vi "ChangePanel.vi"(8 "error in (no error)":errorcluster, 11 "Maui 2.0 in":refnum<class "Maui 2.0.lvclass">) -> (0 "error out":errorcluster, 3 "Maui 2.0 out":refnum<class "Maui 2.0.lvclass">)   [LabVIEW 2020, in "Maui 2.0.lvclass"]
uses:
  Maui 2.0.lvclass
panel:
  in  "Value":i32
  in  "Panel":i32
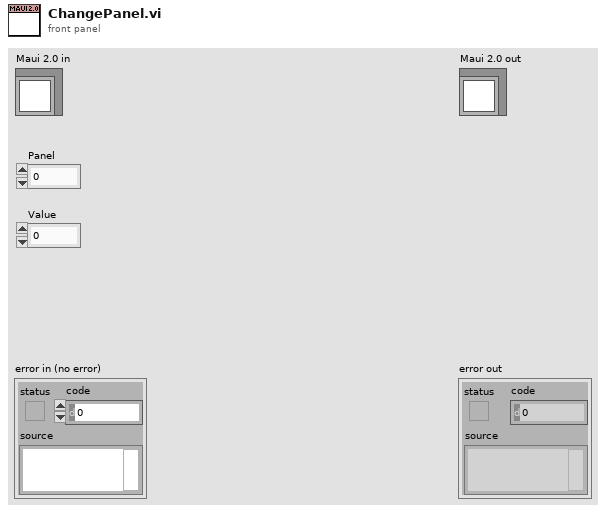
[diagram p1: front panel]
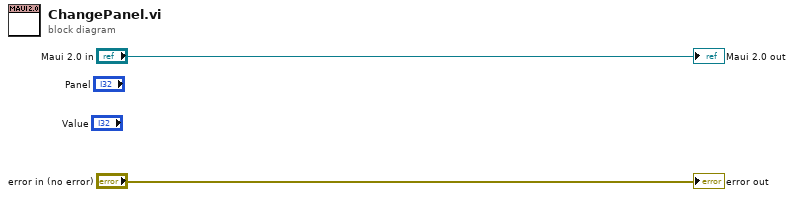
[diagram p0: block diagram]
diagram:
  "error out" <- "error in (no error)"
  "Maui 2.0 out" <- "Maui 2.0 in"
